vi "CheezyAcos.vi"(1 "arg":dbl) -> (0 "acos(arg)":dbl)   [LabVIEW 2015]
uses:
  MathConstantsNames.ctl
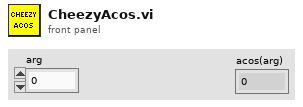
[diagram p1: front panel]
types:
  T1 = typedef "MathConstantsNames.ctl" = enum16{"sq2p1", "sq2m1", "p4", "p3", "p2", "p1", "p0", "q4", "q3", "q2", "q1", "q0", "PIO2"}
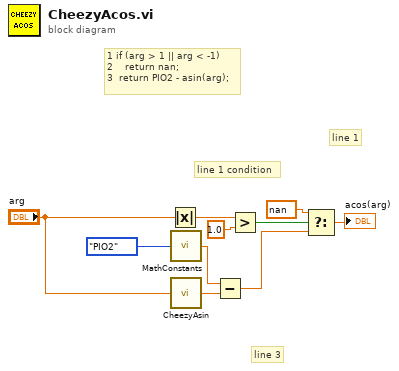
[diagram p0: block diagram]
diagram:
  # "line 3"
  # "line 1"
  # "line 1 condition"
  # "1 if (arg > 1 || arg < -1) \n2    return nan;\n3  return PIO2 - asin(arg);"
  n1 = Absolute Value(x="arg") -> (abs(x)=w10:dbl)
  n2 = call "MathConstants.vi"("Constant Name"=MathConstantsNames."PIO2") -> ("Constant Value"=w4:dbl)
  n3 = call "CheezyAsin.vi"("arg"="arg") -> ("asin(arg)"=w3:dbl)
  n4 = Subtract(x=w4, y=w3) -> (x-y=w2:dbl)
  n5 = Greater?(x=w10, y=1.0) -> (0:w8:bool)
  n6 = Select(t=nan, s=w8, f=w2) -> (s? t:f=→"acos(arg)":dbl)
